vi "CRISTALIZADOR_parametrosMedida.vi"(8 "error in (no error)":errorcluster) -> (0 "error out":errorcluster, 1 "Window":T1={"Nombre ensayo"="Nombre", "Muestra"="Usuario", "Promedios"=10, "Frecuencia adq(s)"=1.0, "Tiempo medida(min) "=0.0} {"Frecuencia adq(s)" format="%.3f"}, 5 "Cancelled?":bool)   [LabVIEW 2017]
doc: "Use this template to create a dialog box with event handling."
uses:
  CRISTALIZADOR_parametrosMedida.ctl
panel:
  in  "Tiempo total (min)":dbl=10.0
  in  "Frecuencia (sec)":dbl=5.0
  in  "Promedios":dbl=1.0
  in  "Muestra":string="Muestra"
  out "HORA":string
  out "FECHA":string
  in  "Ensayo":string="Ensayo"
  in  "Cancel":bool
  in  "OK Button":bool
  # "Datos de la medida"
  # "asslcdms Feb2023 LV17"
  # "( Introduce los datos que aparecen en color azul )"
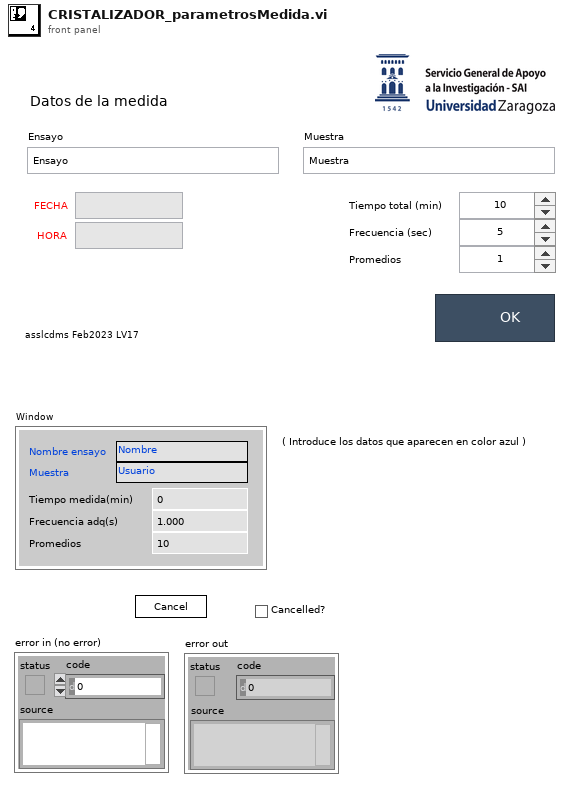
[diagram p1: front panel]
types:
  T1 = typedef "CRISTALIZADOR_parametrosMedida.ctl" = cluster{"Nombre ensayo":string, "Muestra":string, "Promedios":u16, "Frecuencia adq(s)":dbl, "Tiempo medida(min) ":dbl}
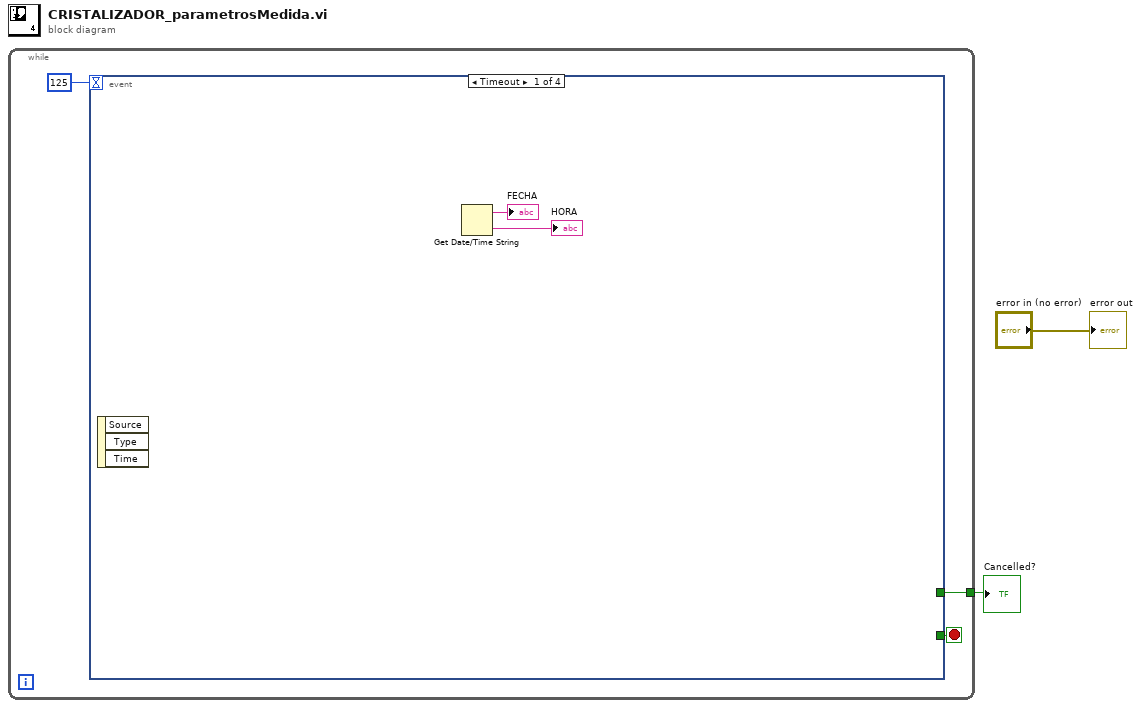
[diagram p0: block diagram]
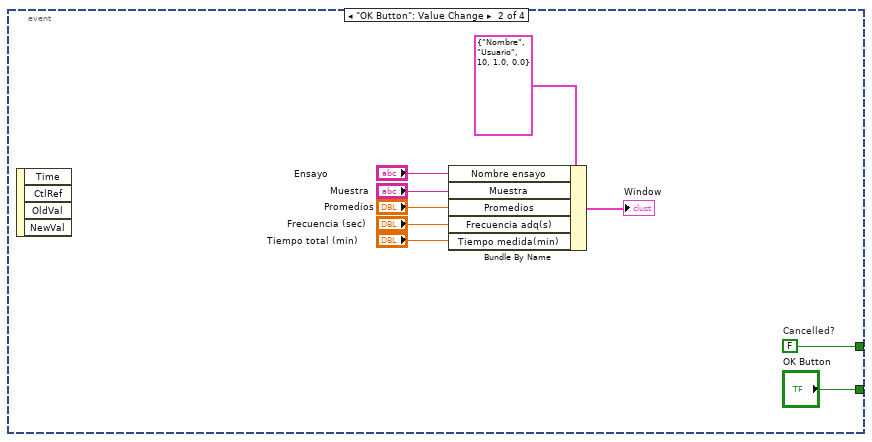
[diagram p2: hidden frame]
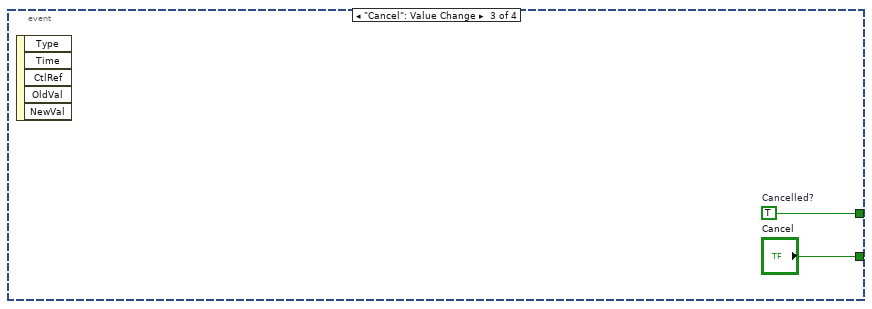
[diagram p3: hidden frame]
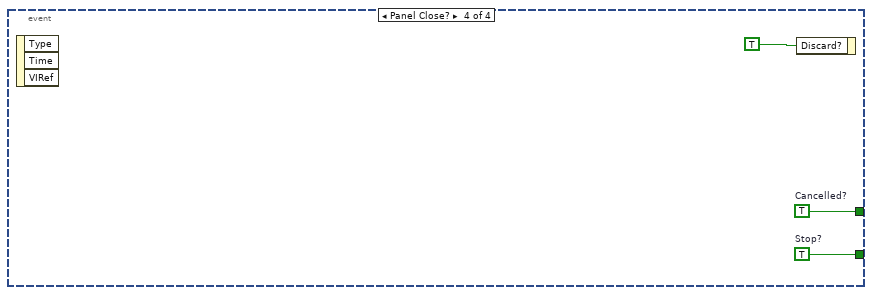
[diagram p4: hidden frame]
diagram:
  n1 = while {
    tunnel: [w4] -> w2
    stop <- w5 stop-if-true
    n2 = event shown="[0] Timeout" {
      selector: _ -> [_ _ _ _]
      dyn-events: _ -> [_ _ _ _]
      timeout: 125 -> [_ _ _ _]
      tunnel: [_ "OK Button" "Cancel" w20] -> w5
      tunnel: [_ w16 w18 w19] -> w4
      event Timeout {
        n3 = event-data() -> ()  [unwired: 1 in, 3 out]
        n4 = Get Date/Time String() -> (date string=→"FECHA":string, time string=→"HORA":string)  [unwired: 3 in]
      }
      event "OK Button": Value Change {
        w16 = FALSE  # Cancelled?
        n5 = event-data() -> ()  [unwired: 1 in, 4 out]
        n6 = Bundle By Name(cluster=T1 {"Nombre ensayo"="Nombre", "Muestra"="Usuario", "Promedios"=10, "Frecuencia adq(s)"=1.0, "Tiempo medida(min) "=0.0} ("Window"), "Nombre ensayo"="Ensayo", "Muestra"="Muestra", "Promedios"="Promedios", "Frecuencia adq(s)"="Frecuencia (sec)", "Tiempo medida(min)"="Tiempo total (min)") -> (→"Window":T1)
      }
      event "Cancel": Value Change {
        w18 = TRUE  # Cancelled?
        n7 = event-data() -> ()  [unwired: 1 in, 5 out]
      }
      event Panel Close? {
        w19 = TRUE  # Cancelled?
        w20 = TRUE  # Stop?
        n8 = event-data() -> ()  [unwired: 1 in, 3 out]
        n9 = event-data("Discard?"=TRUE) -> ()  [unwired: 1 in, 1 out]
      }
    }
  }
  "Cancelled?" <- w2
  "error out" <- "error in (no error)"
